vi "main.vi"() -> ()   [LabVIEW 2010]
uses:
  <vilib>/Platform/TimedLoop/XDataNode/XDataNode.xnode
  <vilib>/Platform/TimedLoop/XDataNode/timing_clust.ctl
  <vilib>/Platform/TimedLoop/XDataNode/nitl_modes.ctl
  <vilib>/Platform/TimedLoop/XDataNode/wakeup.ctl
  <vilib>/eio/EIONode/EIONode.xnode
  <vilib>/rvi/eio/nirviEIOImplementation/nirviEIOImplementation.xnode
  <vilib>/rvi/eio/common/nirviEmuClasses.ctl
  <vilib>/rvi/DataTransferAndStorage/Container/XNode/niFpgaContainer.xnode
  <vilib>/rvi/DataTransferAndStorage/Container/Common/niFpgaContainerMethod.ctl
  <vilib>/rvi/DataTransferAndStorage/Container/Common/niFpgaTransferTypeControl.ctl
  <vilib>/rvi/eio/common/nirviEmuTemplateMethod_noerrors.vi
  <vilib>/rvi/interface/RandomDataEmulation/nirviRandomDataFPGAFIFO.vi
  <vilib>/rvi/interface/RandomDataEmulation/niFpgaRandomDataHandleErrors.vi
  <vilib>/Platform/TimedLoop/XDataNode/XDNodeRunTimeDep.lvlib
panel:
  out "FIFO overflow?":bool
  in  "start":bool
  out "trigger event?":bool
  out "Connector0/DIO36":bool
  out "loop counter":i32
  in  "stop":bool
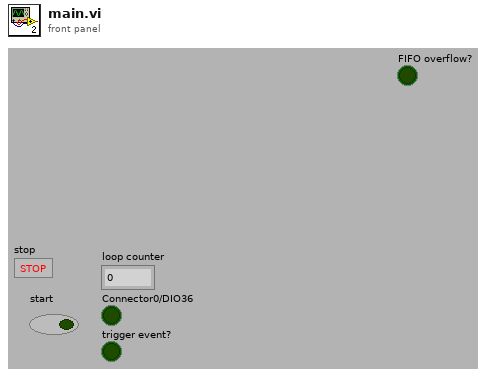
[diagram p1: front panel]
types:
  T1 = typedef "XDNodeRunTimeDep.lvlib/timing_clust.ctl" = cluster{"Expected End [f-1]":u64, "Actual End [f-1]":u64, "Finished Late? [f-1]":bool, "Expected End [i-1]":u64, "Actual End [i-1]":u64, "Finished Late? [i-1]":bool, "Expected Start [i]":u64, "Actual Start [i]":u64, "Expected Start [f]":u64, "Actual Start [f]":u64, "Source Name":string, "Structure Name":string, "Period":i64, "Deadline":i64, "Offset":i64, "Start":i64, "Priority":i32, "Timeout":i32, "Mode":T2, "Wakeup Reason":T3, "Error":errorcluster, "Source Type":string, "Secondary Source Type":string, "Global End Time":u64, "Global Start Time":u64, "Frame Duration":u64, "Iteration Duration":u64, "Assigned CPU":i32, "I/O Scan Engine Mode":u32}
  T2 = typedef "XDNodeRunTimeDep.lvlib/nitl_modes.ctl" = enum32{"No Change", "Process missed periods, maintain original phase", "Discard missed periods, maintain original phase", "Process missed periods, ignore original phase", "Discard missed periods, ignore original phase"}
  T3 = typedef "XDNodeRunTimeDep.lvlib/wakeup.ctl" = enum32{"Normal", "Aborted", "Asynchronous wakeup", "Timing source error", "Timed loop error", "Timeout"}
  T4 = typedef "niFpgaContainerMethod.ctl" = enum16{"<none>", "write", "read", "clear", "getNumberOfElementsToWrite", "getNumberOfElementsToRead", "enable", "disable", "flushAndDisable", "getStreamState", "readA", "readB", "dramWrite", "dramWriteWithByteEnables", "dramRequestData", "dramRetrieveData"}
  T5 = typedef "niFpgaTransferTypeControl.ctl" = enum16{"Target-Scoped", "Host to Target - DMA", "Target to Host - DMA", "Peer to Peer Reader", "Peer to Peer Writer", "Bidirectional"}
  T6 = typedef "nirviEmuClasses.ctl" = enum16{"IO Read", "IO Write", "Method", "Property Read", "Property Write"}
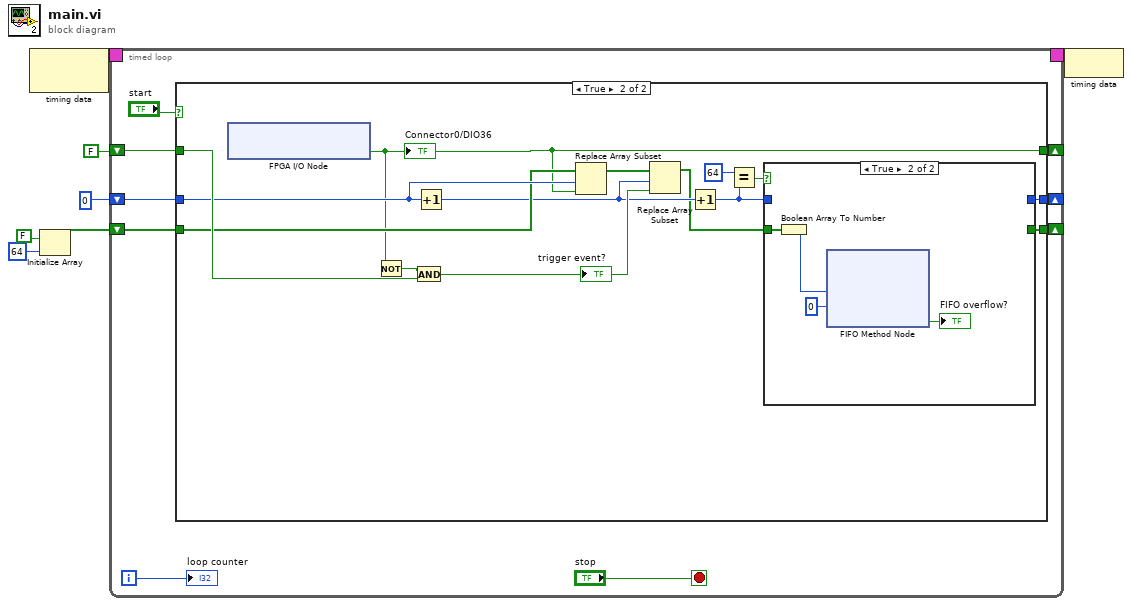
[diagram p0: block diagram]
diagram:
  n1 = node-c288() -> (w7:T1)  [unwired: 1 in]
  n2 = Initialize Array(FALSE, 64 ("dimension size")) -> (w2:bool[])
  n3 = timed-loop {
    timing: w7 -> [_]
    timing-out: [_] -> w6
    shift-right: [w15] -> _
    shift-left: FALSE ("Connector0/DIO36") -> [w16]
    shift-right: [w10] -> _
    shift-left: w2 -> [w11]
    shift-right: [w8] -> _
    shift-left: i16 0 -> [w9]
    i -> [w13]
    stop <- "stop" stop-if-true
    n4 = case shown="True" "start" {
      tunnel: w16 -> [_ w29]
      tunnel: [_ w26] -> w15
      tunnel: w11 -> [_ w27]
      tunnel: [_ w19] -> w10
      tunnel: [_ w17] -> w8
      tunnel: w9 -> [_ w28]
      frame False {
      }
      frame True {
        n5 = xnode "FPGA I/O Node"() -> ("Connector0/DIO36"=w26:bool)  [unwired: 1 in, 1 out]
        "Connector0/DIO36" <- w26
        n6 = Not(x=w26) -> (.not. x?=w30:bool)
        n7 = And(x=w30, y=w29) -> (x .and. y?=w24:bool)
        "trigger event?" <- w24
        n8 = Increment(x=w28) -> (x+1=w23:i16)
        n9 = Replace Array Subset(array=w27, new element=w26, index=w28) -> (w22:bool[])
        n10 = Replace Array Subset(array=w22, new element=w24, index=w23) -> (w20:bool[])
        n11 = Increment(x=w23) -> (x+1=w18:i16)
        n12 = Equal?(x=i16 64, y=w18) -> (x = y?=w21:bool)
        n13 = case shown="True" w21 {
          tunnel: w20 -> [w32 w34]
          tunnel: [w32 _] -> w19
          tunnel: w18 -> [w31 _]
          tunnel: [w31 _] -> w17
          frame False {
          }
          frame True {
            n14 = Boolean Array To Number(Boolean array=w34) -> (number=w33:u64)
            n15 = xnode ("FIFO Method Node")("Element"=w33, "Timeout"=0) -> ("Timed Out?"=→"FIFO overflow?":bool)  [unwired: 1 in, 1 out]
          }
        }
      }
    }
    "loop counter" <- w13
  }
  n16 = node-c288(w6) -> ()
